vi "Write Measurement and Settling Cycles.vi"(0 "signal configuration":refnum<class "SV Function.lvclass">, 5 "measurement cycles":dbl=20.0, 7 "pre-measurement settling cycles":dbl, 9 "post-measurement settling cycles":dbl, 11 "error in (no error)":errorcluster) -> (4 "signal configuration":refnum<class "SV Function.lvclass">, 15 "error out":errorcluster)   [LabVIEW 2017, in "SV Function.lvclass"]
uses:
  <vilib>/addons/_NISVFA/_Generation/Signal Generation/SV Function/SV Function.lvclass
  <vilib>/addons/_NISVFA/_Generation/Signal Generation/SV Function/SV Function.lvclass/SV Function.ctl
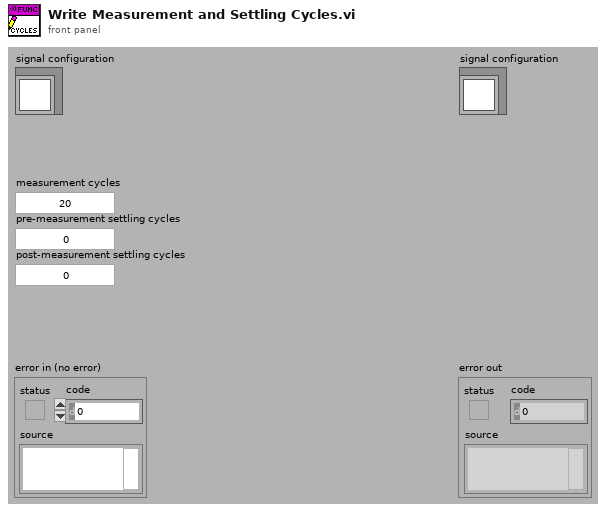
[diagram p1: front panel]
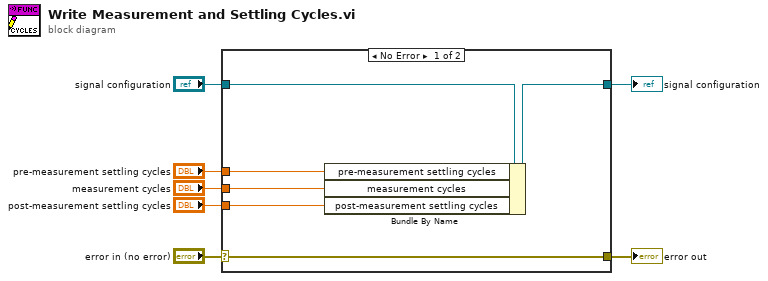
[diagram p0: block diagram]
diagram:
  n1 = case shown="No Error" "error in (no error)" {
    selector: "error in (no error)" -> [w13 w14]
    tunnel: [w13 w14] -> w6
    tunnel: [w11 w15] -> w4
    tunnel: "signal configuration" -> [w12 w15]
    tunnel: "pre-measurement settling cycles" -> [w10 _]
    tunnel: "measurement cycles" -> [w9 _]
    tunnel: "post-measurement settling cycles" -> [w8 _]
    frame No Error {
      n2 = Bundle By Name(cluster=w12, "pre-measurement settling cycles"=w10, "measurement cycles"=w9, "post-measurement settling cycles"=w8) -> (w11:refnum<class "SV Function.lvclass">)
    }
    frame Error {
    }
  }
  "error out" <- w6
  "signal configuration" <- w4
